vi "Insight_Profile_Avaliable.vi"(8 "error in (no error)":errorcluster, 11 "telnet connection":T1) -> (0 "error out":errorcluster, 1 "commands":string[](array[string]), 2 "response data":string, 3 "telnet  connection out":T1)   [LabVIEW 2015]
doc: "Insight Photonic Solutions\n\nQueries the instrument for the avalable custom power profiles. The avalable profiles are returned as a string array.\n\nver 1.0 - original release\n\nInput:\nTelnet connection\nError in\n\nOutput:\nTelnet connection\nError Out\nCommands (Command Array)\nResponse Data"
uses:
  Telnet Session.ctl
  <vilib>/Utility/error.llb/whitespace.ctl
  <vilib>/regexp/Match Regular Expression.xnode
panel:
  out "whole match":string
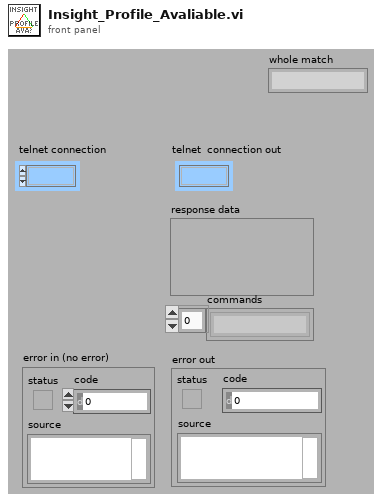
[diagram p1: front panel]
types:
  T1 = typedef "Telnet Session.ctl" = refnum<k1>
  T2 = typedef "whitespace.ctl" = u16
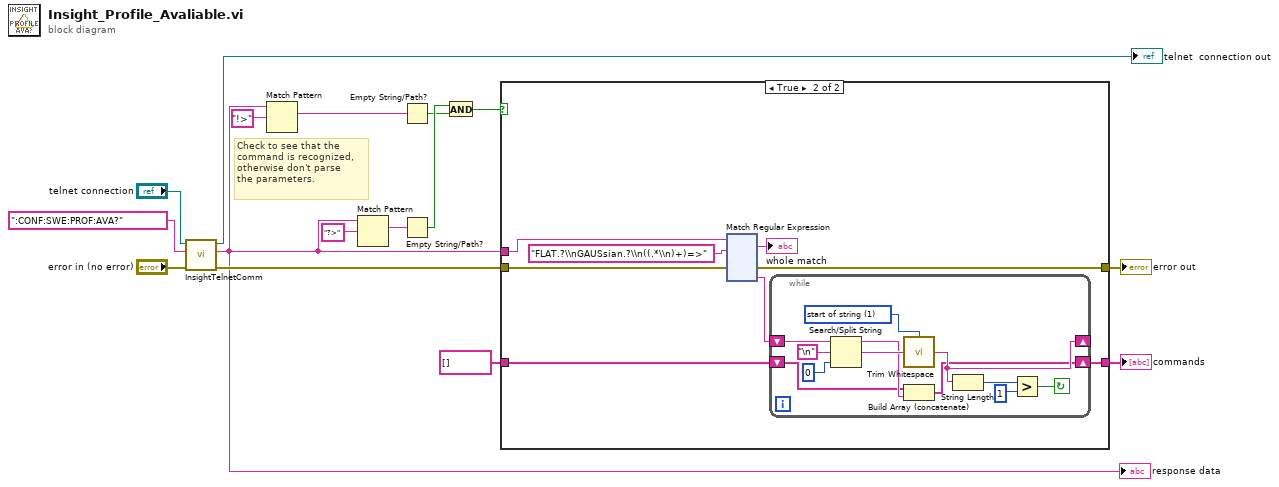
[diagram p0: block diagram]
diagram:
  # "Check to see that the \ncommand is recognized,\notherwise don't parse \nthe parameters."
  n1 = call "InsightTelnetComm.vi"("error in"="error in (no error)", "write buffer (\"\")"=":CONF:SWE:PROF:AVA?" ("String"), "telnet connection"="telnet connection") -> ("error out"=w16:errorcluster, "response data"=w6:string, "telnet  connection out"=→"telnet  connection out":T1)  [unwired: 4 in]
  "response data" <- w6
  n2 = Match Pattern(string=w6, regular expression="!>") -> (match substring=w11:string)  [unwired: 1 in, 3 out]
  n3 = Match Pattern(string=w6, regular expression="?>") -> (match substring=w12:string)  [unwired: 1 in, 3 out]
  n4 = Empty String/Path?(string/path=w11) -> (empty?=w8:bool)
  n5 = Empty String/Path?(string/path=w12) -> (empty?=w9:bool)
  n6 = And(x=w9, y=w8) -> (x .and. y?=w7:bool)
  n7 = case shown="True" w7 {
    tunnel: [w18 w22] -> w5
    tunnel: w16 -> [w18 w23]
    tunnel: w6 -> [_ w24]
    tunnel: [w17 w21] -> w4
    tunnel: string[] [] ("array") -> [w17 w20]
    frame False {
    }
    frame True {
      n8 = xnode "Match Regular Expression"("input string"=w24, "regular expression"="FLAT.?\\nGAUSsian.?\\n((.*\\n)+)=>", "error in"=w23) -> ("whole match"=→"whole match":string, "error out"=w22:errorcluster, "submatch 1"=w25:string)  [unwired: 3 in, 3 out]
      n9 = while {
        shift-right: [w31] -> _
        shift-left: w25 -> [w38]
        shift-right: [w29] -> w21
        shift-left: w20 -> [w28]
        stop <- w34 continue-if-true
        w33 = T2 1 items=["both", "start of string", "end of string"] ("location (both)")
        n10 = Search/Split String(string=w38, search string/char (-)="\n", offset (0)=0) -> (substring before match=w30:string, match + rest of string=w32:string)  [unwired: 1 out]
        n11 = call <vilib>:"Trim Whitespace.vi"("string"=w32, "location (both)"=w33) -> ("trimmed string"=w31:string)
        n12 = Build Array (concatenate)(w28, w30) -> (w29:string[])
        n13 = String Length(string=w31) -> (length=w36:i32)
        n14 = Greater?(x=w36, y=1) -> (0:w34:bool)
      }
    }
  }
  "error out" <- w5
  "commands" <- w4
